vi "READ CAN.vi"(7 "STATES":T1=enum."CLOSE COMM") -> ()   [LabVIEW 2018]
uses:
  <vilib>/xnet/xnet.llb/XNET Frame CAN.ctl
  <vilib>/xnet/xnet.llb/XNET Frame Type CAN.ctl
  CONTROLS/STATES.ctl
  <resource>/objmgr/xnet.rc
  <vilib>/xnet/xnet.llb/XNET Create Session (Frame Output Stream).vi
  <vilib>/xnet/xnet.llb/XNET Write (Frame CAN).vi
panel:
  in  "data":T2[](array[typedef])=[{"timestamp"=timestamp(0 s since 1904-01-01), "payload"=[1, 2, 3, 4, 5, 6, 7, 8], "identifier"=2, "type"=0, "extended?"=FALSE, "echo?"=FALSE}, {"timestamp"=timestamp(0 s since 1904-01-01), "payload"=[0, 1, 2, 3, 4, 5, 6, 7], "identifier"=3, "type"=0, "extended?"=FALSE, "echo?"=FALSE}] {"payload" format="%x"; "timestamp" format="%<%.7X\n%x>T"; "type" items=["CAN Data"=0, "CAN Remote"=1, "CAN Bus Error"=2, "CAN 2.0 Data"=8, "CAN FD Data"=16, "CAN FD+BRS Data"=24, "J1939 Data"=192, "Delay"=224, "Log Trigger"=225, "Start Trigger"=226]; "identifier" format="%x"}
  in  "CAN Cluster 2":refnum<k21>=":memory:"
  in  "Interface Baud Rate":u32=125000
  in  "Select Interface 2":refnum<k21>="CAN1"
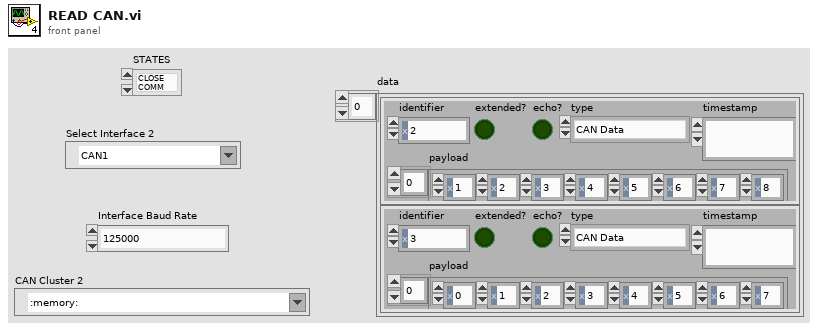
[diagram p1: front panel]
types:
  T1 = typedef "STATES.ctl" = enum16{"OPEN COMM", "WRITE FRAME", "CLOSE COMM"}
  T2 = typedef "XNET Frame CAN.ctl" = cluster{"timestamp":timestamp, "payload":u8[], "identifier":u32, "type":T3, "extended?":bool, "echo?":bool}
  T3 = typedef "XNET Frame Type CAN.ctl" = u8
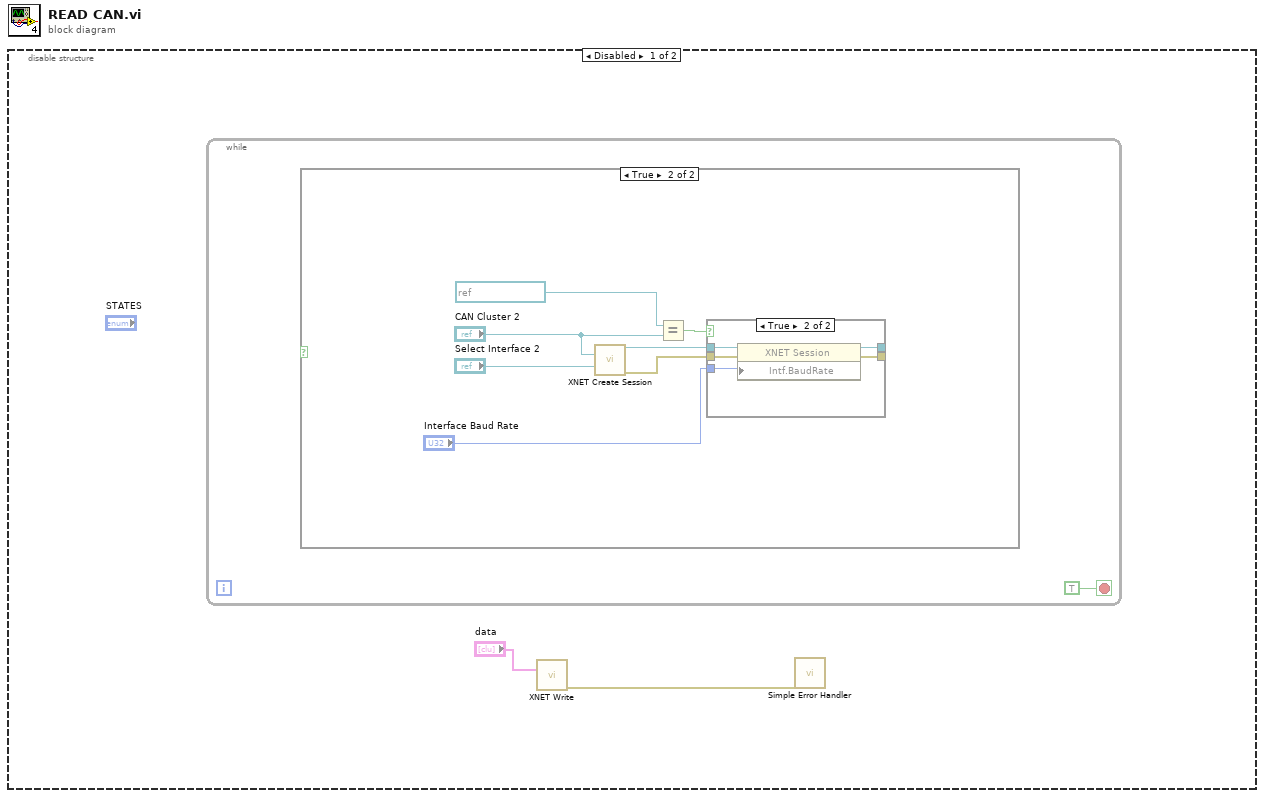
[diagram p0: block diagram]
diagram:
  n1 = disable-structure shown="Disabled" {
    frame Disabled {
      n2 = while {
        stop <- TRUE stop-if-true
        n3 = case shown="True" {
          selector: _ -> [_ _]
          frame False {
          }
          frame True {
            n4 = call-poly <vilib>:"XNET Create Session.vi"("cluster (:memory:)"="CAN Cluster 2", "interface"="Select Interface 2") -> ("session out"=w9:refnum<k21>, "error out"=w7:errorcluster)  [unwired: 1 in, 11 out]
            n5 = Equal?(x=refnum<k21> ":memory:" ("CAN Cluster"), y="CAN Cluster 2") -> (x = y?=w4:bool)
            n6 = case shown="True" w4 {
              tunnel: w9 -> [w12 w17]
              tunnel: [w12 w16] -> _
              tunnel: "Interface Baud Rate" -> [_ w15]
              tunnel: [w11 w14] -> _
              tunnel: w7 -> [w11 w13]
              frame False {
              }
              frame True {
                n7 = property class="XNET Session"(reference=w17, error in=w13, "Intf.BaudRate"=w15) -> (reference out=w16:refnum<k21>, error out=w14:errorcluster)
              }
            }
          }
        }
      }
      n8 = call-poly <vilib>:"XNET Write.vi"("data"="data") -> ("error out"=w2:errorcluster)  [unwired: 2 in, 12 out]
      n9 = call <vilib>:"Simple Error Handler.vi"("error in (no error)"=w2) -> ()  [unwired: 1 in, 8 out]
    }
    frame Enabled {
    }
  }
